vi "Measurement Test.vi"(8 "error in (no error)":errorcluster, 9 "Channel":string, 10 "Position":u32, 11 "Measurement":refnum<class "Measurement.lvclass">) -> (0 "error out":errorcluster, 3 "Passed":bool)   [LabVIEW 2015, in "Measurement.lvclass"]
uses:
  Measurement.lvclass
  Driver Test/Driver Test.lvclass
  Test Class/Test Class.lvclass
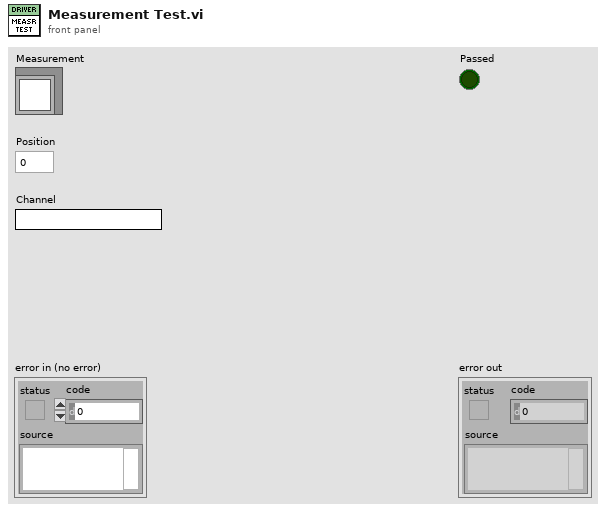
[diagram p1: front panel]
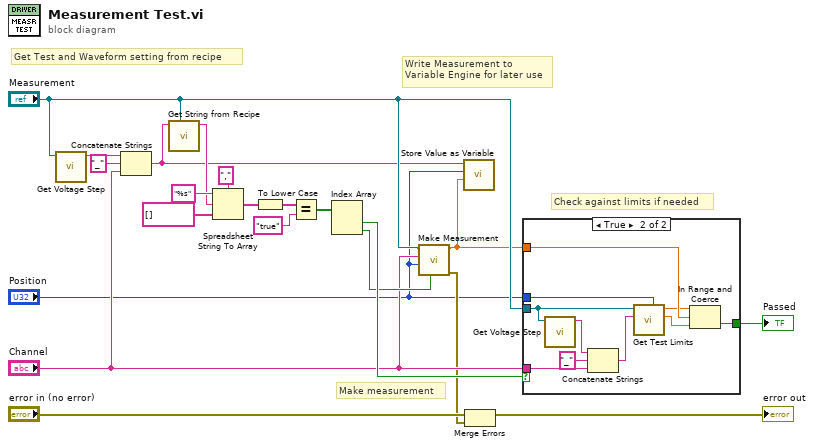
[diagram p0: block diagram]
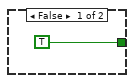
[diagram p2: hidden frame]
diagram:
  # "Check against limits if needed"
  # "Write Measurement to \nVariable Engine for later use"
  # "Make measurement"
  # "Get Test and Waveform setting from recipe"
  n1 = call "Get Voltage Step.vi"("Driver Test in"="Measurement") -> ("Voltage Step"=w6:string)  [unwired: 9 in, 1 out]
  n2 = Concatenate Strings(w6, "_" ("element"), "Channel") -> (w3:string)
  n3 = call "Get String from Recipe.vi"("Test Class in"="Measurement", "Name"=w3) -> ("Value"=w4:string)  [unwired: 7 in, 2 out]
  n4 = Spreadsheet String To Array(delimiter (Tab)=",", format string="%s", spreadsheet string=w4, array type (2D Dbl)=string[] []) -> (array=w16:string[])
  n5 = To Lower Case(string=w16) -> (all lower case string=w17:string[])
  n6 = Equal?(x=w17, y="true") -> (x = y?=w19:bool[])
  n7 = Index Array(array=w19) -> (element #1=w20:bool, element #2=w11:bool)  [unwired: 2 in]
  n8 = call "Make Measurement.vi"("Full Waveform"=w11, "Position"="Position", "Channel"="Channel", "Driver Test in"="Measurement") -> ("error out"=w7:errorcluster, "Value"=w1:dbl)  [unwired: 6 in]
  n9 = call "Store Value as Variable.vi"("Value"=w1, "Position"="Position", "Variable Name"=w3) -> ()  [unwired: 9 in]
  n10 = Merge Errors("error in (no error)", w7) -> (→"error out":errorcluster)
  n11 = case shown="True" w20 {
    tunnel: "Measurement" -> [_ w27]
    tunnel: "Channel" -> [_ w24]
    tunnel: [TRUE w32] -> w9
    tunnel: w1 -> [_ w31]
    tunnel: "Position" -> [_ w30]
    frame False {
    }
    frame True {
      n12 = call "Get Voltage Step.vi"("Driver Test in"=w27) -> ("Voltage Step"=w25:string)  [unwired: 9 in, 1 out]
      n13 = Concatenate Strings(w25, "_" ("string"), w24) -> (w23:string)
      n14 = call "Get Test Limits.vi"("Position"=w30, "Channel"=w23, "Test Class in"=w27) -> ("Lower Limit"=w28:dbl, "Upper Limit"=w29:dbl)  [unwired: 6 in, 1 out]
      n15 = In Range and Coerce(upper limit=w29, x=w31, lower limit=w28) -> (In Range?=w32:bool)  [unwired: 1 out]
    }
  }
  "Passed" <- w9
